vi "Save To XML.vi"(7 "include size in file name? (F)":bool, 8 "error in":errorcluster, 9 "duplicate names warning? (T)":bool=TRUE, 10 "layout keyword":string, 11 "state in":T1) -> (0 "error out":errorcluster, 3 "state out":T1)   [LabVIEW 2010, in "NI_SE_Config Front Panel Layout.lvlib"]
uses:
  NI_SE_Config Front Panel Layout.lvlib
  State.ctl
  VI Info.ctl
  VI Panel Layout/VI Panel Layout.lvclass
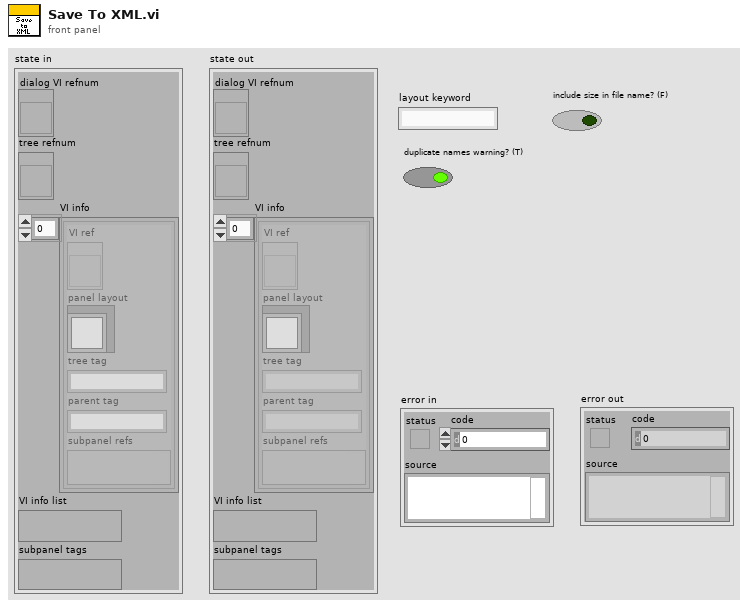
[diagram p1: front panel]
types:
  T1 = typedef "NI_SE_Config Front Panel Layout.lvlib/State.ctl" = cluster{"dialog VI refnum":refnum<vi>, "tree refnum":refnum<vi>, "VI info":T2[], "VI info list":variant, "subpanel tags":variant}
  T2 = typedef "NI_SE_Config Front Panel Layout.lvlib/VI Info.ctl" = cluster{"VI ref":refnum<vi>, "panel layout":refnum<class "VI Panel Layout.lvclass">, "tree tag":string, "parent tag":string, "subpanel refs":variant}
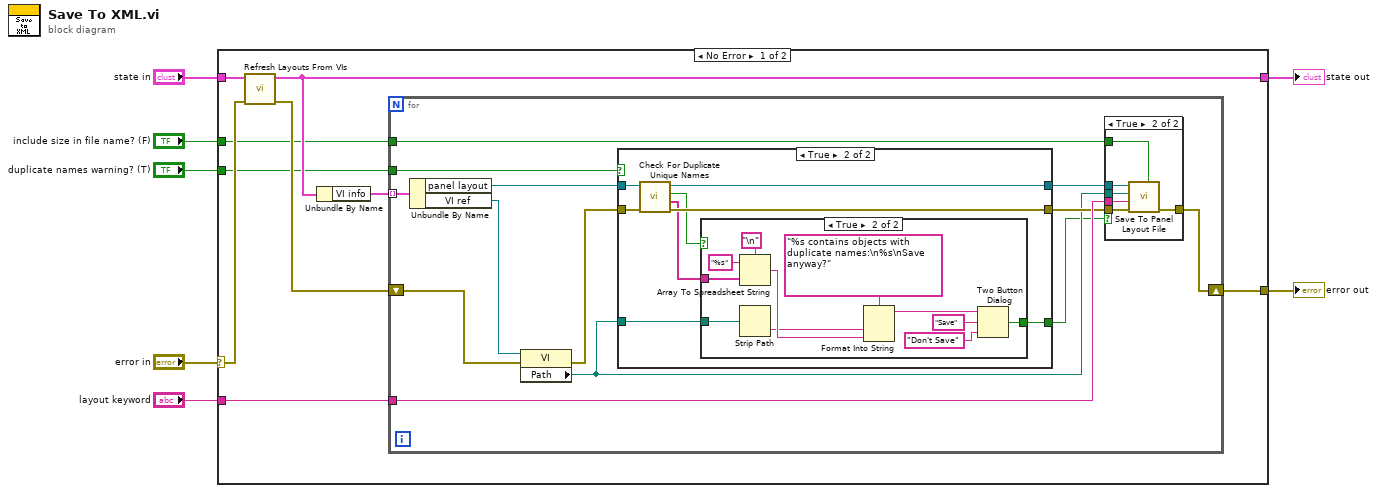
[diagram p0: block diagram]
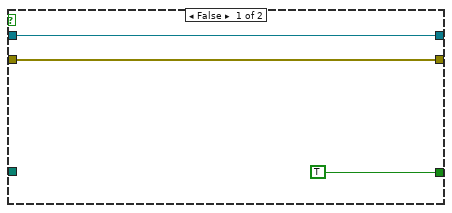
[diagram p3: hidden frame]
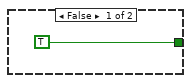
[diagram p4: hidden frame]
diagram:
  n1 = case shown="No Error" "error in" {
    selector: "error in" -> [w12 w61]
    tunnel: "state in" -> [w13 w60]
    tunnel: [w14 w61] -> w6
    tunnel: "layout keyword" -> [w16 _]
    tunnel: [w10 w60] -> w3
    tunnel: "duplicate names warning? (T)" -> [w9 _]
    tunnel: "include size in file name? (F)" -> [w8 _]
    frame No Error {
      n2 = call "Refresh Layouts From VIs.vi"("error in"=w12, "state in"=w13) -> ("error out"=w11:errorcluster, "state out"=w10:T1)  [unwired: 8 in]
      n3 = Unbundle By Name(w10) -> ("VI info"=w15:T2[])
      n4 = for {
        tunnel: w15 -> [w29] mode=indexing
        tunnel: w16 -> [w28]
        shift-right: [w26] -> w14
        shift-left: w11 -> [w27]
        tunnel: w9 -> [w20]
        tunnel: w8 -> [w17]
        n5 = Unbundle By Name(w29) -> ("panel layout"=w24:refnum<class "VI Panel Layout.lvclass">, "VI ref"=w25:refnum<vi>)
        n6 = property class="VI"(reference=w25, error in=w27) -> (error out=w22:errorcluster, "Path"=w19:path)  [unwired: 1 out]
        n7 = case shown="True" w20 {
          tunnel: w24 -> [w39 w47]
          tunnel: [w39 w46] -> w23
          tunnel: w22 -> [w38 w45]
          tunnel: [w38 w44] -> w21
          tunnel: w19 -> [_ w41]
          tunnel: [TRUE ("T button?") w40] -> w18
          frame False {
          }
          frame True {
            n8 = call "Check For Duplicate Unique Names.vi"("error in (no error)"=w45, "VI Panel Layout in"=w47) -> ("error out"=w44:errorcluster, "duplicate names"=w42:string[], "duplicates found?"=w43:bool, "VI Panel Layout out"=w46:refnum<class "VI Panel Layout.lvclass">)  [unwired: 6 in]
            n9 = case shown="True" w43 {
              tunnel: w42 -> [_ w59]
              tunnel: w41 -> [_ w54]
              tunnel: [TRUE ("T button?") w49] -> w40
              frame False {
              }
              frame True {
                n10 = Array To Spreadsheet String(delimiter (Tab)="\n", array=w59, 3:"%s" ("format string")) -> (spreadsheet string=w56:string)
                n11 = Strip Path(path=w54) -> (name=w53:string)  [unwired: 1 out]
                n12 = Format Into String(format string="%s contains objects with duplicate names:\n%s\nSave anyway?", w53, w56) -> (resulting string=w52:string)  [unwired: 2 in, 1 out]
                n13 = Two Button Dialog(message=w52, 1:"Don't Save" ("F button name (\"Cancel\")"), 2:"Save" ("T button name (\"OK\")")) -> (T button?=w49:bool)
              }
            }
          }
        }
        n14 = case shown="True" w18 {
          tunnel: w28 -> [_ w36]
          tunnel: [w30 w35] -> w26
          tunnel: w23 -> [_ w34]
          tunnel: w21 -> [w30 w33]
          tunnel: w19 -> [_ w32]
          tunnel: w17 -> [_ w31]
          frame False {
          }
          frame True {
            n15 = call "Save To Panel Layout File.vi"("include size in file name? (F)"=w31, "error in)"=w33, "layout keyword (\"\")"=w36, "VI path"=w32, "panel layout in"=w34) -> ("error out"=w35:errorcluster)  [unwired: 4 in, 2 out]
          }
        }
      }
    }
    frame Error {
    }
  }
  "state out" <- w3
  "error out" <- w6
